vi "Introspection Core.vi"(8 "error in (no error)":errorcluster, 11 "CS++Fgen in":refnum<class "CS++Fgen.lvclass">) -> (0 "error out":errorcluster, 2 "CS++Messages":refnum<class "Message.lvclass">[](array[class]), 3 "CS++Fgen out":refnum<class "CS++Fgen.lvclass">)   [LabVIEW 2016, in "CS++Fgen.lvlib" / "CS++Fgen.lvclass"]
doc: "This vi delivers a list with all messages this actor reacts to. \n\nNote that all inherited classes have to overwrite it."
uses:
  CS++Fgen.lvclass
  <vilib>/ActorFramework/Message/Message.lvclass
  CS++Fgen Messages/Abort Generation Msg/Abort Generation Msg.lvclass
  C:/Program Files (x86)/National Instruments/LabVIEW 2016/vi.lib/ActorFramework/Message/Message.lvclass
  CS++Fgen Messages/Clear Arbitrary Memory [SEQ] Msg/Clear Arbitrary Memory [SEQ] Msg.lvclass
  CS++Fgen Messages/Clear Arbitrary Sequence [SEQ] Msg/Clear Arbitrary Sequence [SEQ] Msg.lvclass
  CS++Fgen Messages/Clear Arbitrary Waveform [ARB] Msg/Clear Arbitrary Waveform [ARB] Msg.lvclass
  CS++Fgen Messages/Configure Advanced Trigger [AT] Msg/Configure Advanced Trigger [AT] Msg.lvclass
  CS++Fgen Messages/Configure AM Enabled [AM] Msg/Configure AM Enabled [AM] Msg.lvclass
  CS++Fgen Messages/Configure AM Internal [AM] Msg/Configure AM Internal [AM] Msg.lvclass
  CS++Fgen Messages/Configure AM Source [AM] Msg/Configure AM Source [AM] Msg.lvclass
  CS++Fgen Messages/Configure Arb Frequency [AF] Msg/Configure Arb Frequency [AF] Msg.lvclass
  CS++Fgen Messages/Configure Arbitrary Sequence [SEQ] Msg/Configure Arbitrary Sequence [SEQ] Msg.lvclass
  CS++Fgen Messages/Configure Arbitrary Waveform [ARB] Msg/Configure Arbitrary Waveform [ARB] Msg.lvclass
  CS++Fgen Messages/Configure Burst Count [BST] Msg/Configure Burst Count [BST] Msg.lvclass
  CS++Fgen Messages/Configure Data Marker [DM] Msg/Configure Data Marker [DM] Msg.lvclass
  CS++Fgen Messages/Configure FM Enabled [FM] Msg/Configure FM Enabled [FM] Msg.lvclass
  CS++Fgen Messages/Configure FM Internal [FM] Msg/Configure FM Internal [FM] Msg.lvclass
  CS++Fgen Messages/Configure FM Source [FM] Msg/Configure FM Source [FM] Msg.lvclass
  CS++Fgen Messages/Configure Internal Trigger Rate [IT] Msg/Configure Internal Trigger Rate [IT] Msg.lvclass
  CS++Fgen Messages/Configure Operation Mode Msg/Configure Operation Mode Msg.lvclass
  CS++Fgen Messages/Configure Output Enable Msg/Configure Output Enable Msg.lvclass
  CS++Fgen Messages/Configure Output Impedance Msg/Configure Output Impedance Msg.lvclass
  CS++Fgen Messages/Configure Output Mode Msg/Configure Output Mode Msg.lvclass
  CS++Fgen Messages/Configure Ref Clock Source Msg/Configure Ref Clock Source Msg.lvclass
  CS++Fgen Messages/Configure Resume Trigger [RT] Msg/Configure Resume Trigger [RT] Msg.lvclass
  CS++Fgen Messages/Configure Sample Clock [SC] Msg/Configure Sample Clock [SC] Msg.lvclass
  CS++Fgen Messages/Configure Sample Clock Output Enabled [SC] Msg/Configure Sample Clock Output Enabled [SC] Msg.lvclass
  CS++Fgen Messages/Configure Sample Rate [ARB] Msg/Configure Sample Rate [ARB] Msg.lvclass
  CS++Fgen Messages/Configure Sparse Marker [SM] Msg/Configure Sparse Marker [SM] Msg.lvclass
  CS++Fgen Messages/Configure Standard Waveform [STD] Msg/Configure Standard Waveform [STD] Msg.lvclass
  CS++Fgen Messages/Configure Start Trigger [STT] Msg/Configure Start Trigger [STT] Msg.lvclass
  CS++Fgen Messages/Configure Stop Trigger [SPT] Msg/Configure Stop Trigger [SPT] Msg.lvclass
  CS++Fgen Messages/Configure Trigger Source [TRG] Msg/Configure Trigger Source [TRG] Msg.lvclass
  CS++Fgen Messages/Create Arbitrary Sequence [SEQ] Msg/Create Arbitrary Sequence [SEQ] Msg.lvclass
  CS++Fgen Messages/Create Arbitrary Waveform [ARB] Msg/Create Arbitrary Waveform [ARB] Msg.lvclass
  CS++Fgen Messages/Create Channel Arbitrary Waveform [ACH] Msg/Create Channel Arbitrary Waveform [ACH] Msg.lvclass
  CS++Fgen Messages/Create Channel Arbitrary Waveform I16 [ACH] Msg/Create Channel Arbitrary Waveform I16 [ACH] Msg.lvclass
  CS++Fgen Messages/Create Channel Arbitrary Waveform I32 [ACH] Msg/Create Channel Arbitrary Waveform I32 [ACH] Msg.lvclass
  CS++Fgen Messages/Disable All Data Markers [DM] Msg/Disable All Data Markers [DM] Msg.lvclass
  CS++Fgen Messages/Disable All Sparse Markers [SM] Msg/Disable All Sparse Markers [SM] Msg.lvclass
  CS++Fgen Messages/Get Channel Name Msg/Get Channel Name Msg.lvclass
  CS++Fgen Messages/Get Data Marker Name [DM] Msg/Get Data Marker Name [DM] Msg.lvclass
  CS++Fgen Messages/Get Sparse Marker Indexes [SM] Msg/Get Sparse Marker Indexes [SM] Msg.lvclass
  CS++Fgen Messages/Get Sparse Marker Name [SM] Msg/Get Sparse Marker Name [SM] Msg.lvclass
  CS++Fgen Messages/Initiate Generation Msg/Initiate Generation Msg.lvclass
  CS++Fgen Messages/Query Arb Sequence Capabilities [SEQ] Msg/Query Arb Sequence Capabilities [SEQ] Msg.lvclass
  CS++Fgen Messages/Query Arb Waveform Capabilities 64 [ARB64] Msg/Query Arb Waveform Capabilities 64 [ARB64] Msg.lvclass
  CS++Fgen Messages/Query Arb Waveform Capabilities [ARB] Msg/Query Arb Waveform Capabilities [ARB] Msg.lvclass
  CS++Fgen Messages/Send Software Advanced Trigger [AT] Msg/Send Software Advanced Trigger [AT] Msg.lvclass
  CS++Fgen Messages/Send Software Hold Trigger [HT] Msg/Send Software Hold Trigger [HT] Msg.lvclass
  CS++Fgen Messages/Send Software Resume Trigger [RT] Msg/Send Software Resume Trigger [RT] Msg.lvclass
  CS++Fgen Messages/Send Software Stop Trigger [SPT] Msg/Send Software Stop Trigger [SPT] Msg.lvclass
  CS++Fgen Messages/Send Software Trigger [TRG] Msg/Send Software Trigger [TRG] Msg.lvclass
  CS++Fgen Messages/Set Sparse Marker Indexes [SM] Msg/Set Sparse Marker Indexes [SM] Msg.lvclass
  CSPP_Core/Actors/CS++DeviceActor/CS++DeviceActor.lvclass
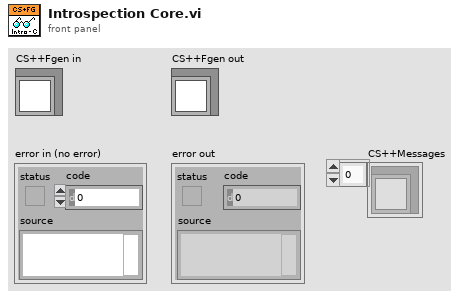
[diagram p1: front panel]
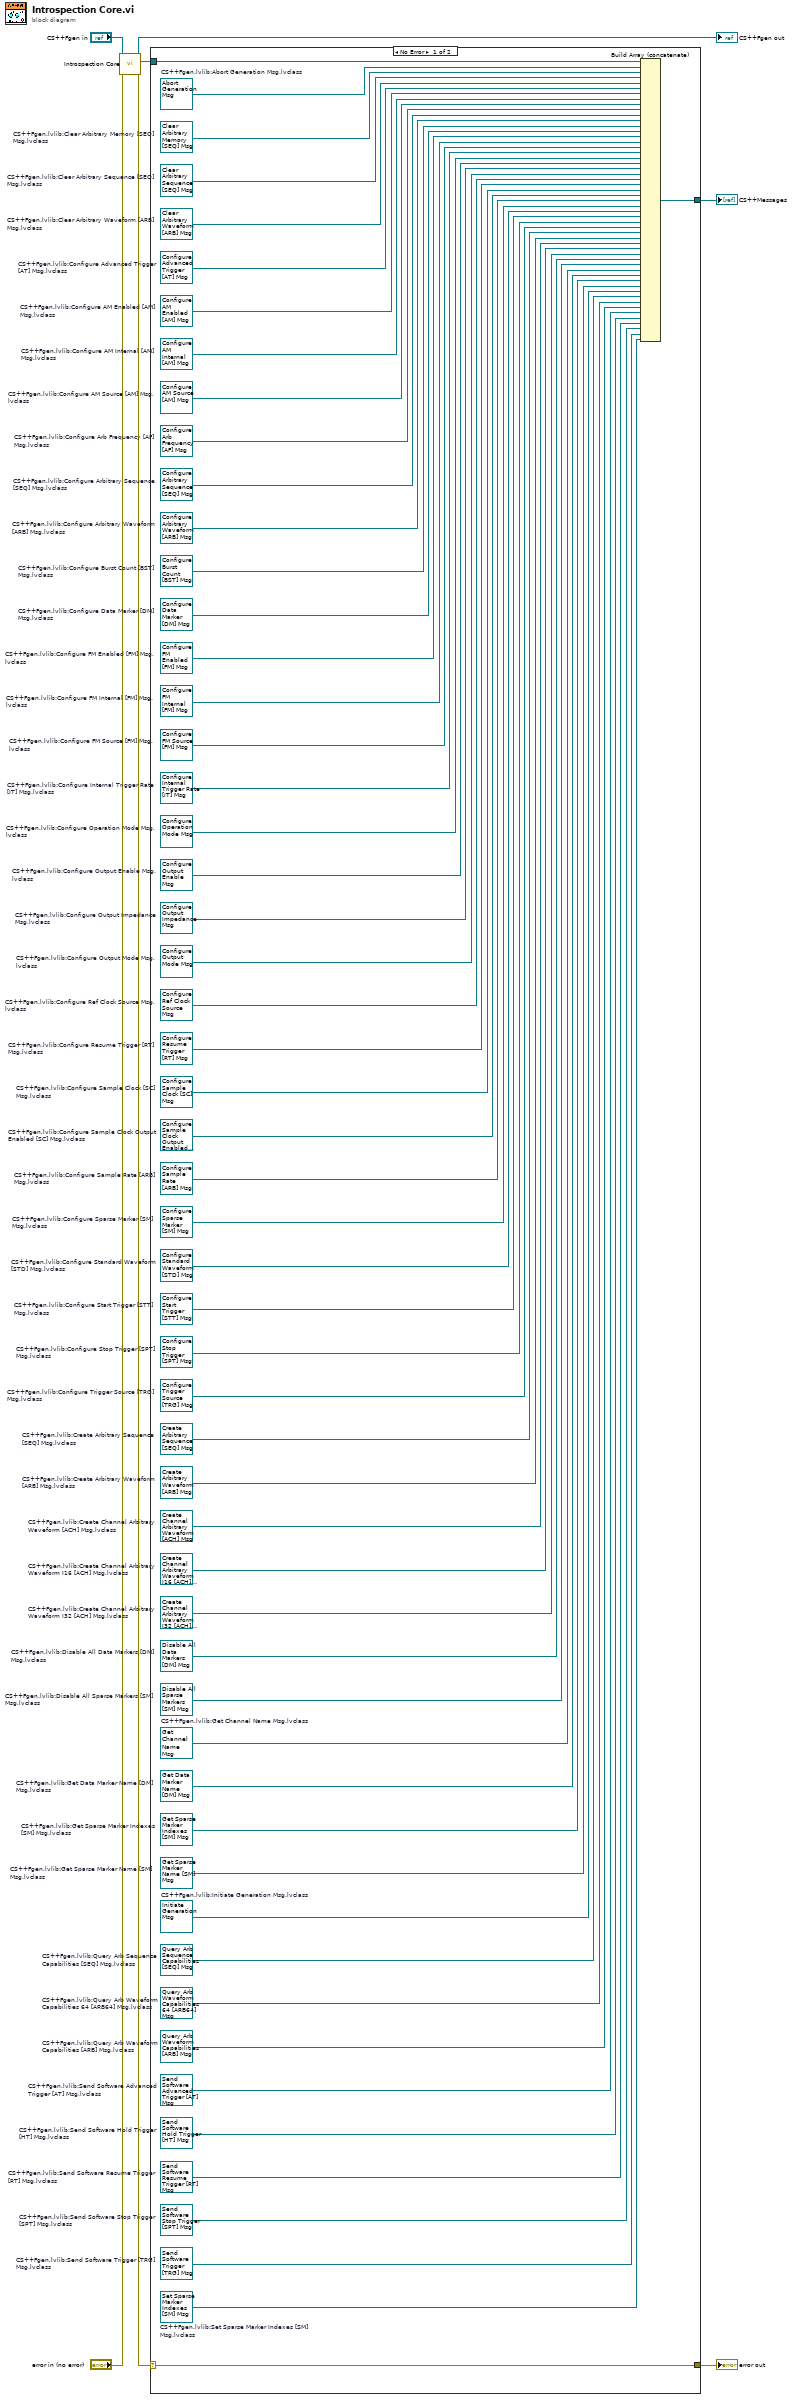
[diagram p0: block diagram]
diagram:
  n1 = call-parent "Introspection Core.vi"("error in (no error)"="error in (no error)", "CS++DeviceActor in"="CS++Fgen in") -> ("error out"=w4:errorcluster, "CS++Messages"=w2:refnum<class "Message.lvclass">[], "CS++DeviceActor out"=→"CS++Fgen out":refnum<class "CS++Fgen.lvclass">)  [unwired: 7 in]
  n2 = case shown="No Error" w4 {
    selector: w4 -> [w62 w63]
    tunnel: [w62 w63] -> w3
    tunnel: w2 -> [w61 _]
    tunnel: [w8 _] -> w1
    frame No Error {
      w9 = refnum<class "Set Sparse Marker Indexes [SM] Msg.lvclass"> refnum  # CS++Fgen.lvlib:Set Sparse Marker Indexes [SM] Msg.lvclass
      w10 = refnum<class "Send Software Trigger [TRG] Msg.lvclass"> refnum  # CS++Fgen.lvlib:Send Software Trigger [TRG] Msg.lvclass
      w11 = refnum<class "Send Software Stop Trigger [SPT] Msg.lvclass"> refnum  # CS++Fgen.lvlib:Send Software Stop Trigger [SPT] Msg.lvclass
      w12 = refnum<class "Send Software Resume Trigger [RT] Msg.lvclass"> refnum  # CS++Fgen.lvlib:Send Software Resume Trigger [RT] Msg.lvclass
      w13 = refnum<class "Send Software Hold Trigger [HT] Msg.lvclass"> refnum  # CS++Fgen.lvlib:Send Software Hold Trigger [HT] Msg.lvclass
      w14 = refnum<class "Send Software Advanced Trigger [AT] Msg.lvclass"> refnum  # CS++Fgen.lvlib:Send Software Advanced Trigger [AT] Msg.lvclass
      w15 = refnum<class "Query Arb Waveform Capabilities [ARB] Msg.lvclass"> refnum  # CS++Fgen.lvlib:Query Arb Waveform Capabilities [ARB] Msg.lvclass
      w16 = refnum<class "Query Arb Waveform Capabilities 64 [ARB64] Msg.lvclass"> refnum  # CS++Fgen.lvlib:Query Arb Waveform Capabilities 64 [ARB64] Msg.lvclass
      w17 = refnum<class "Query Arb Sequence Capabilities [SEQ] Msg.lvclass"> refnum  # CS++Fgen.lvlib:Query Arb Sequence Capabilities [SEQ] Msg.lvclass
      w18 = refnum<class "Initiate Generation Msg.lvclass"> refnum  # CS++Fgen.lvlib:Initiate Generation Msg.lvclass
      w19 = refnum<class "Get Sparse Marker Name [SM] Msg.lvclass"> refnum  # CS++Fgen.lvlib:Get Sparse Marker Name [SM] Msg.lvclass
      w20 = refnum<class "Get Sparse Marker Indexes [SM] Msg.lvclass"> refnum  # CS++Fgen.lvlib:Get Sparse Marker Indexes [SM] Msg.lvclass
      w21 = refnum<class "Get Data Marker Name [DM] Msg.lvclass"> refnum  # CS++Fgen.lvlib:Get Data Marker Name [DM] Msg.lvclass
      w22 = refnum<class "Get Channel Name Msg.lvclass"> refnum  # CS++Fgen.lvlib:Get Channel Name Msg.lvclass
      w23 = refnum<class "Disable All Sparse Markers [SM] Msg.lvclass"> refnum  # CS++Fgen.lvlib:Disable All Sparse Markers [SM] Msg.lvclass
      w24 = refnum<class "Disable All Data Markers [DM] Msg.lvclass"> refnum  # CS++Fgen.lvlib:Disable All Data Markers [DM] Msg.lvclass
      w25 = refnum<class "Create Channel Arbitrary Waveform I32 [ACH] Msg.lvclass"> refnum  # CS++Fgen.lvlib:Create Channel Arbitrary Waveform I32 [ACH] Msg.lvclass
      w26 = refnum<class "Create Channel Arbitrary Waveform I16 [ACH] Msg.lvclass"> refnum  # CS++Fgen.lvlib:Create Channel Arbitrary Waveform I16 [ACH] Msg.lvclass
      w27 = refnum<class "Create Channel Arbitrary Waveform [ACH] Msg.lvclass"> refnum  # CS++Fgen.lvlib:Create Channel Arbitrary Waveform [ACH] Msg.lvclass
      w28 = refnum<class "Create Arbitrary Waveform [ARB] Msg.lvclass"> refnum  # CS++Fgen.lvlib:Create Arbitrary Waveform [ARB] Msg.lvclass
      w29 = refnum<class "Create Arbitrary Sequence [SEQ] Msg.lvclass"> refnum  # CS++Fgen.lvlib:Create Arbitrary Sequence [SEQ] Msg.lvclass
      w30 = refnum<class "Configure Trigger Source [TRG] Msg.lvclass"> refnum  # CS++Fgen.lvlib:Configure Trigger Source [TRG] Msg.lvclass
      w31 = refnum<class "Configure Stop Trigger [SPT] Msg.lvclass"> refnum  # CS++Fgen.lvlib:Configure Stop Trigger [SPT] Msg.lvclass
      w32 = refnum<class "Configure Start Trigger [STT] Msg.lvclass"> refnum  # CS++Fgen.lvlib:Configure Start Trigger [STT] Msg.lvclass
      w33 = refnum<class "Configure Standard Waveform [STD] Msg.lvclass"> refnum  # CS++Fgen.lvlib:Configure Standard Waveform [STD] Msg.lvclass
      w34 = refnum<class "Configure Sparse Marker [SM] Msg.lvclass"> refnum  # CS++Fgen.lvlib:Configure Sparse Marker [SM] Msg.lvclass
      w35 = refnum<class "Configure Sample Rate [ARB] Msg.lvclass"> refnum  # CS++Fgen.lvlib:Configure Sample Rate [ARB] Msg.lvclass
      w36 = refnum<class "Configure Sample Clock Output Enabled [SC] Msg.lvclass"> refnum  # CS++Fgen.lvlib:Configure Sample Clock Output Enabled [SC] Msg.lvclass
      w37 = refnum<class "Configure Sample Clock [SC] Msg.lvclass"> refnum  # CS++Fgen.lvlib:Configure Sample Clock [SC] Msg.lvclass
      w38 = refnum<class "Configure Resume Trigger [RT] Msg.lvclass"> refnum  # CS++Fgen.lvlib:Configure Resume Trigger [RT] Msg.lvclass
      w39 = refnum<class "Configure Ref Clock Source Msg.lvclass"> refnum  # CS++Fgen.lvlib:Configure Ref Clock Source Msg.lvclass
      w40 = refnum<class "Configure Output Mode Msg.lvclass"> refnum  # CS++Fgen.lvlib:Configure Output Mode Msg.lvclass
      w41 = refnum<class "Configure Output Impedance Msg.lvclass"> refnum  # CS++Fgen.lvlib:Configure Output Impedance Msg.lvclass
      w42 = refnum<class "Configure Output Enable Msg.lvclass"> refnum  # CS++Fgen.lvlib:Configure Output Enable Msg.lvclass
      w43 = refnum<class "Configure Operation Mode Msg.lvclass"> refnum  # CS++Fgen.lvlib:Configure Operation Mode Msg.lvclass
      w44 = refnum<class "Configure Internal Trigger Rate [IT] Msg.lvclass"> refnum  # CS++Fgen.lvlib:Configure Internal Trigger Rate [IT] Msg.lvclass
      w45 = refnum<class "Configure FM Source [FM] Msg.lvclass"> refnum  # CS++Fgen.lvlib:Configure FM Source [FM] Msg.lvclass
      w46 = refnum<class "Configure FM Internal [FM] Msg.lvclass"> refnum  # CS++Fgen.lvlib:Configure FM Internal [FM] Msg.lvclass
      w47 = refnum<class "Configure FM Enabled [FM] Msg.lvclass"> refnum  # CS++Fgen.lvlib:Configure FM Enabled [FM] Msg.lvclass
      w48 = refnum<class "Configure Data Marker [DM] Msg.lvclass"> refnum  # CS++Fgen.lvlib:Configure Data Marker [DM] Msg.lvclass
      w49 = refnum<class "Configure Burst Count [BST] Msg.lvclass"> refnum  # CS++Fgen.lvlib:Configure Burst Count [BST] Msg.lvclass
      w50 = refnum<class "Configure Arbitrary Waveform [ARB] Msg.lvclass"> refnum  # CS++Fgen.lvlib:Configure Arbitrary Waveform [ARB] Msg.lvclass
      w51 = refnum<class "Configure Arbitrary Sequence [SEQ] Msg.lvclass"> refnum  # CS++Fgen.lvlib:Configure Arbitrary Sequence [SEQ] Msg.lvclass
      w52 = refnum<class "Configure Arb Frequency [AF] Msg.lvclass"> refnum  # CS++Fgen.lvlib:Configure Arb Frequency [AF] Msg.lvclass
      w53 = refnum<class "Configure AM Source [AM] Msg.lvclass"> refnum  # CS++Fgen.lvlib:Configure AM Source [AM] Msg.lvclass
      w54 = refnum<class "Configure AM Internal [AM] Msg.lvclass"> refnum  # CS++Fgen.lvlib:Configure AM Internal [AM] Msg.lvclass
      w55 = refnum<class "Configure AM Enabled [AM] Msg.lvclass"> refnum  # CS++Fgen.lvlib:Configure AM Enabled [AM] Msg.lvclass
      w56 = refnum<class "Configure Advanced Trigger [AT] Msg.lvclass"> refnum  # CS++Fgen.lvlib:Configure Advanced Trigger [AT] Msg.lvclass
      w57 = refnum<class "Clear Arbitrary Waveform [ARB] Msg.lvclass"> refnum  # CS++Fgen.lvlib:Clear Arbitrary Waveform [ARB] Msg.lvclass
      w58 = refnum<class "Clear Arbitrary Sequence [SEQ] Msg.lvclass"> refnum  # CS++Fgen.lvlib:Clear Arbitrary Sequence [SEQ] Msg.lvclass
      w59 = refnum<class "Clear Arbitrary Memory [SEQ] Msg.lvclass"> refnum  # CS++Fgen.lvlib:Clear Arbitrary Memory [SEQ] Msg.lvclass
      w60 = refnum<class "Abort Generation Msg.lvclass"> refnum  # CS++Fgen.lvlib:Abort Generation Msg.lvclass
      n3 = Build Array (concatenate)(w61, w60, w59, w58, w57, w56, w55, w54, w53, w52, w51, w50, w49, w48, w47, w46, w45, w44, w43, w42, w41, w40, w39, w38, w37, w36, w35, w34, w33, w32, w31, w30, w29, w28, w27, w26, w25, w24, w23, w22, w21, w20, w19, w18, w17, w16, w15, w14, w13, w12, w11, w10, w9) -> (w8:refnum<class "Message.lvclass">[])
    }
    frame Error {
    }
  }
  "error out" <- w3
  "CS++Messages" <- w1
